vi "MorphologyCore.vi"(5 "MorphologyType":T1, 6 "Iterations":u16, 7 "Anchor Point":T2={"x"=-1, "y"=-1}, 8 "error in (no error)":errorcluster, 9 "Structuring Element":bool[][](array[boolean]), 10 "Morphology Result":T3, 11 "Greyscale Image-Source":T3) -> (0 "error out":errorcluster)   [LabVIEW 2020, in "g_ar_toolkit.image.lvlib"]
uses:
  g_ar_toolkit.image.lvlib
  g_ar_toolkit.common/g_ar_toolkit.common.lvlib
  Greyscale Image.ctl
  g_ar_toolkit.common/Image Point (Integer).ctl
  MorphologyTypes.ctl
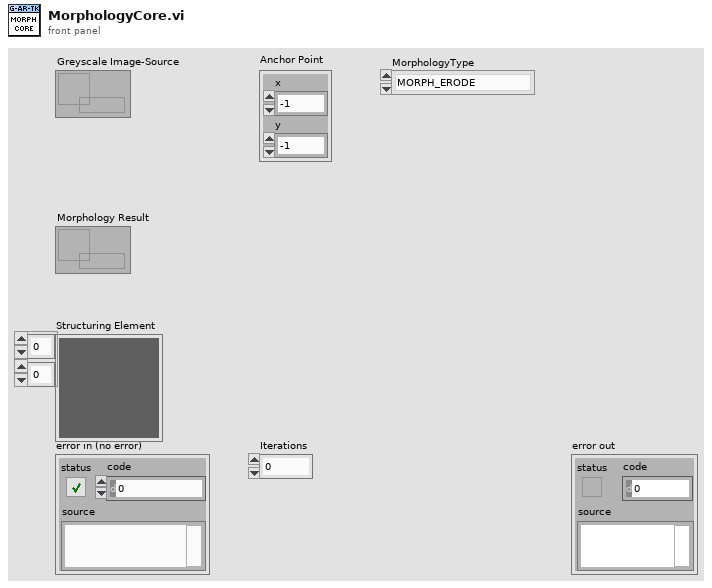
[diagram p1: front panel]
types:
  T1 = typedef "g_ar_toolkit.image.lvlib/MorphologyTypes.ctl" = enum16{"MORPH_ERODE", "MORPH_DILATE", "MORPH_OPEN", "MORPH_CLOSE", "MORPH_GRADIENT", "MORPH_TOPHAT", "MORPH_BLACKHAT", "MORPH_HITMISS"}
  T2 = typedef "g_ar_toolkit.common.lvlib/Image Point (Integer).ctl" = cluster{"x":i32, "y":i32}
  T3 = typedef "g_ar_toolkit.image.lvlib/Greyscale Image.ctl" = refnum<data-value>
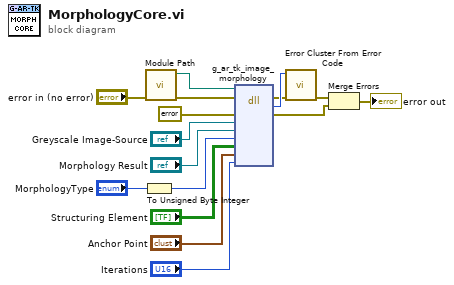
[diagram p0: block diagram]
diagram:
  n1 = To Unsigned Byte Integer(number="MorphologyType") -> (unsigned 8bit integer=w5:u8)
  n2 = call "Module Path.vi"("error in (no error)"="error in (no error)") -> ("error out"=w7:errorcluster, "Path"=w6:path)  [unwired: 9 in]
  n3 = dll-call lib="?" fn="g_ar_tk_image_morphology" ("g_ar_toolkit.*.*:g_ar_tk_image_in_range")(path in=w6, error in=w7, "error_cluster"=errorcluster {"status"=FALSE, "code"=0, "source"=""} ("error constant"), "EDVR src"="Greyscale Image-Source", "EDVR dst"="Morphology Result", "operation"=w5, "kernel"="Structuring Element", "anchor_point"="Anchor Point", "iterations"="Iterations") -> (error out=w8:errorcluster, "MgErr"=w9:i32, "error_cluster"=w12:errorcluster)  [unwired: 7 in, 1 out]
  n4 = call <vilib>:"Error Cluster From Error Code.vi"("error in (no error)"=w8, "error code (0)"=w9) -> ("error out"=w10:errorcluster)  [unwired: 7 in]
  n5 = Merge Errors(w10, w12) -> (→"error out":errorcluster)
